vi "wavelength scan_v2.0.vi"() -> ()   [LabVIEW 2012]
panel:
  out "HSRLTEC_offset":dbl=0.01321159999999999 format="%#.4g"
  in  "HSRL_offset":dbl=0.0132 format="%.4g"
  out "Readings":T1={"Pro8000"=TRUE, "WV OnLine TEC"=23.1576786, "WV Online TEC"=TRUE, "WV Online LD"=0.175435558, "WV Online LD"=TRUE, "WV Offline TEC"=29.527338, "WV Offline TEC"=TRUE, "WV Offline LD"=0.175292984, "WV Offline LD"=TRUE, "WV EtalonTEC"=31.6442299, "WV Etalon TEC"=TRUE, "HSRL Etalon TEC"=25.9487457, "HSRL Etalon TEC"=TRUE, "HSRL TEC"=14.2976322, "HSRL TEC "=TRUE, "HSRL LD"=0.160083994, "HSRL LD"=TRUE} {"HSRL LD" format="%.3p"; "HSRL TEC" format="%.3g"; "WV Offline LD" format="%.3p"; "WV Online LD" format="%.3p"; "HSRL Etalon TEC" format="%.3g"; "WV EtalonTEC" format="%.3g"; "WV Offline TEC" format="%.3g"; "WV OnLine TEC" format="%.3g"}
  in  "Settings":T2={"Module"=enum."HSRL TEC", "WV Online TEC"=23.15274999999951, "WV Online LD"=0.175, "WV Offline TEC"=29.514, "WV Offline LD"=0.175, "WV Etalon TEC"=30.61, "HSRL Etalon TEC"=25.954, "HSRL TEC"=14.022, "HSRL LD"=0.16} {"HSRL LD" min=0.0 max=0.18 step=0.001 format="%.3p"; "HSRL TEC" min=14.0 max=28.0 step=0.1 format="%.3g"; "WV Offline LD" min=0.0 max=0.18 step=0.001 format="%.3p"; "WV Online LD" min=0.0 max=0.18 step=0.001 format="%.3p"; "HSRL Etalon TEC" format="%.2g"; "WV Etalon TEC" format="%.2g"; "WV Offline TEC" min=16.0 max=30.0 step=0.1 format="%.3g"; "WV Online TEC" min=14.0 max=28.0 step=0.1 format="%.3g"}
  in  "channel\n0 WV online,\n1, WVoffline\n2, HSRL":i32=2
  out "Power Chart":dbl(graph)=0.0001022
  in  "range (0=auto)":i32
  in  "wavelength":i32=4
  in  "filter (0=out)":i32
  out "OfflineTEC_offset":dbl=0.013673700000001787 format="%#.4g"
  out "OnLineTEC_offset":dbl=0.007064800000488702 format="%.4g"
  in  "WV OnlineTEC_offset":dbl format="%.4g"
  in  "WV OfflineTEC_offset":dbl format="%.4g"
  out "Lambda Read (nm)":dbl=780.2608711081949 format="%.5f"
  out "Wavelength Lock":bool=TRUE
  out "XY Graph":cluster{"Y":dbl[], "Y":dbl[]}[](graph)
  out "Power (W)":dbl=0.0001022 format="%.3p"
  out "OphirPM":T3={"Ophir-Ref"=refnum, "Ophir-Device"=1000, "Ophir-Channel"=0}
  out "Waveform Chart":dbl(graph)=780.2608711081949
  in  "Lambda Step (nm)":dbl=5e-05 format="%.5f"
  in  "Lambda Stop (nm)":dbl=780.261 format="%.5f"
  in  "Lambda Start (nm)":dbl=780.231 format="%.5f"
  in  "step_size":dbl=0.0015 format="%#_6p"
  in  "Device In":refnum<visa-resource-name>="GPIB0::10::INSTR"
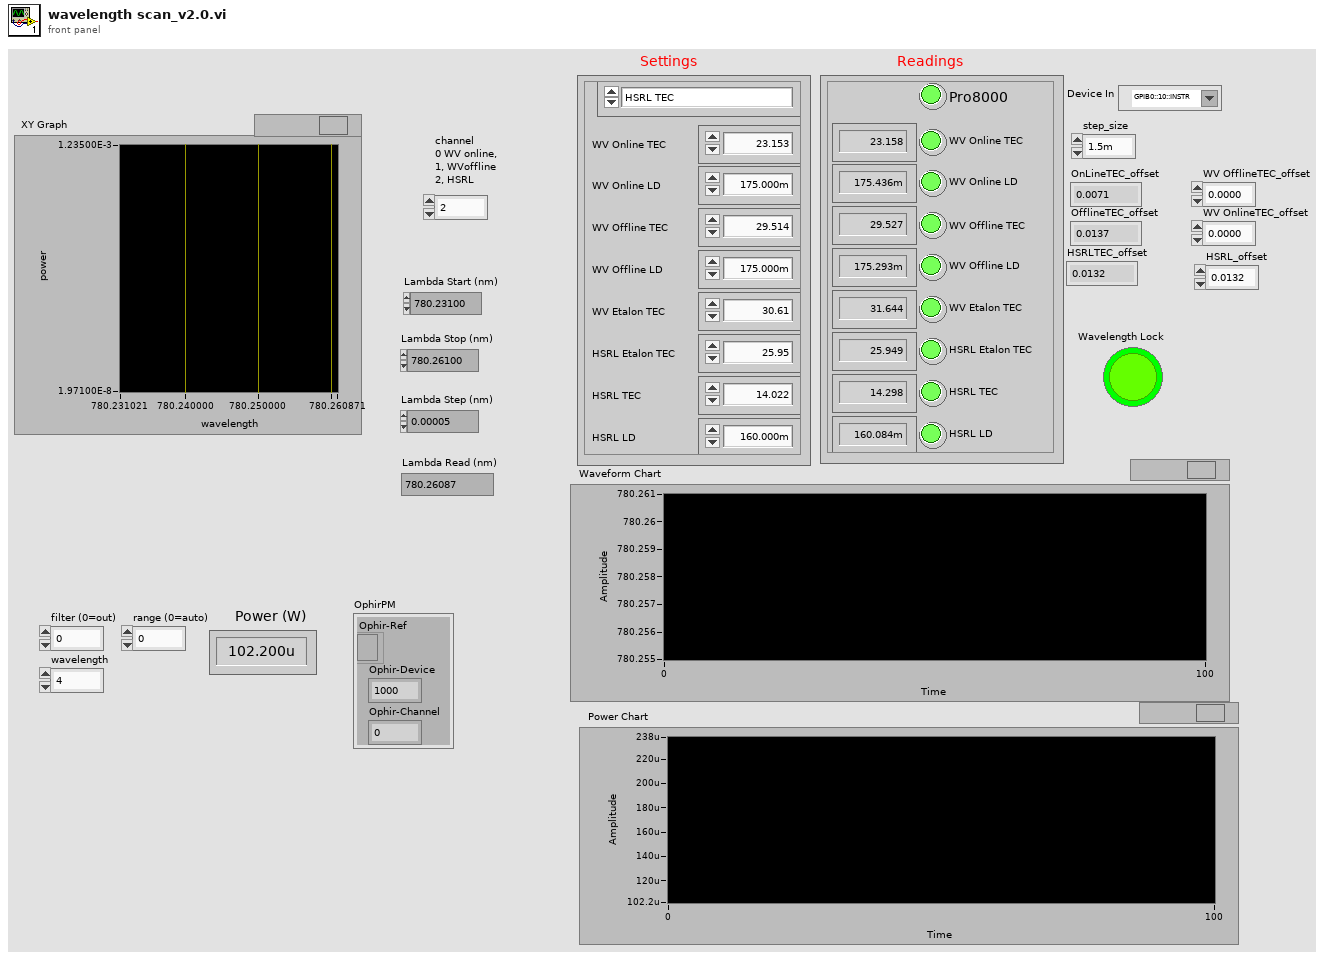
[diagram p1: front panel]
types:
  T1 = cluster{"Pro8000":bool, "WV OnLine TEC":dbl, "WV Online TEC":bool, "WV Online LD":dbl, "WV Online LD":bool, "WV Offline TEC":dbl, "WV Offline TEC":bool, "WV Offline LD":dbl, "WV Offline LD":bool, "WV EtalonTEC":dbl, "WV Etalon TEC":bool, "HSRL Etalon TEC":dbl, "HSRL Etalon TEC":bool, "HSRL TEC":dbl, "HSRL TEC ":bool, "HSRL LD":dbl, "HSRL LD":bool}
  T2 = cluster{"Module":enum16{"WV Online TEC", "WV Online LD", "WV Offline TEC", "WV Offline LD", "WV Etalon TEC", "HSRL Etalon TEC", "HSRL TEC", "HSRL LD"}, "WV Online TEC":dbl, "WV Online LD":dbl, "WV Offline TEC":dbl, "WV Offline LD":dbl, "WV Etalon TEC":dbl, "HSRL Etalon TEC":dbl, "HSRL TEC":dbl, "HSRL LD":dbl}
  T3 = cluster{"Ophir-Ref":refnum<k7>, "Ophir-Device":i32, "Ophir-Channel":i32}
  T4 = enum16{"WV Online TEC", "WV Online LD", "WV Offline TEC", "WV Offline LD", "WV Etalon TEC", "HSRL Etalon TEC", "HSRL TEC", "HSRL LD"}
  T5 = enum16{"Open_TL", "Close_TL", "Verify_ID", "TEC_Sensor", "SET", "READ", "ON", "OFF", "Set_Limits", "Read_Limits", "Enable_Status", "Read_Status"}
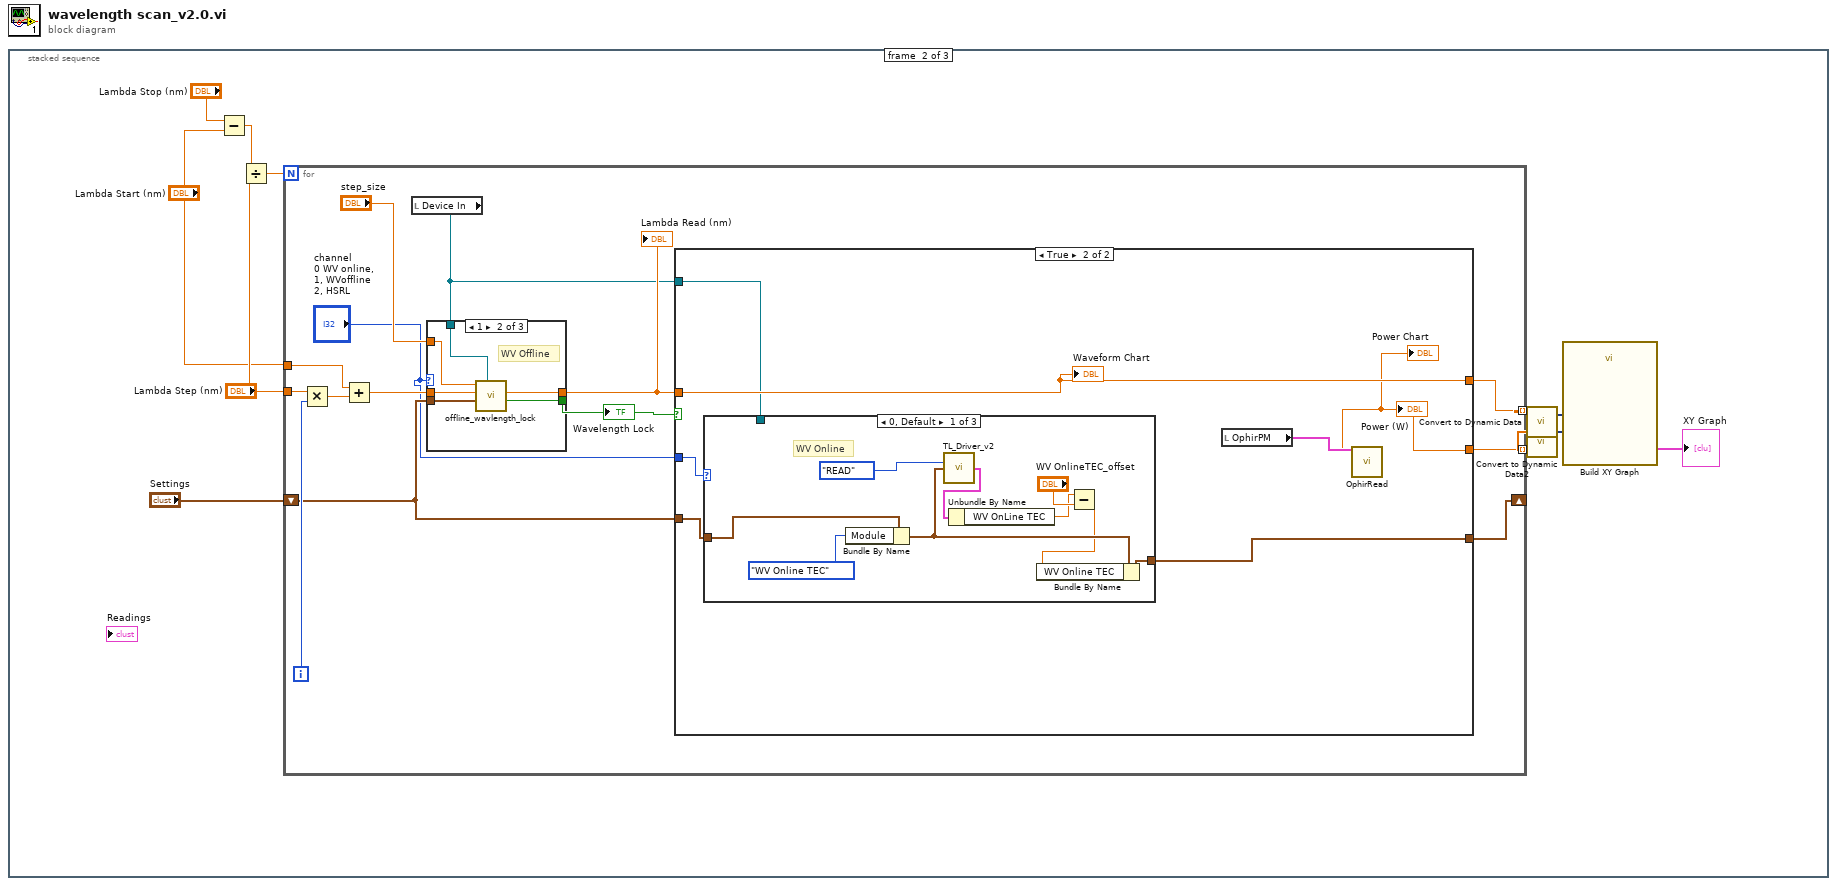
[diagram p0: block diagram]
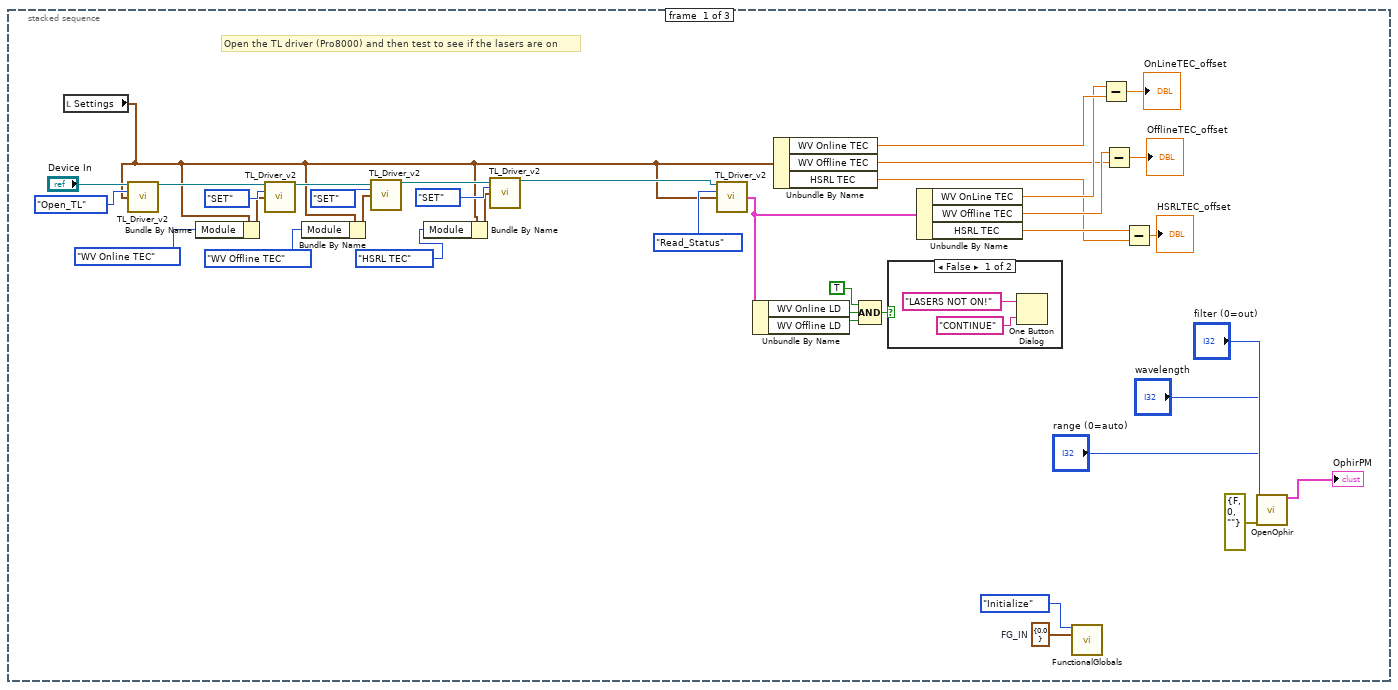
[diagram p2: hidden frame]
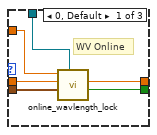
[diagram p4: hidden frame]
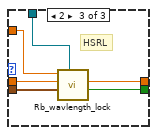
[diagram p5: hidden frame]
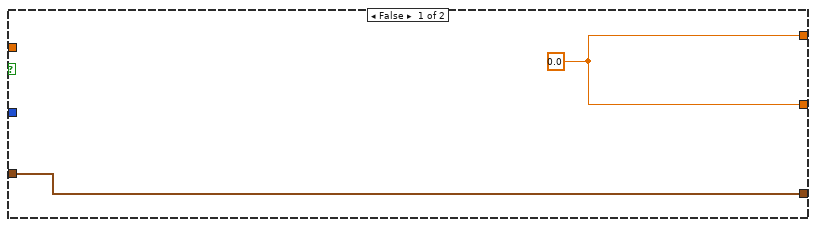
[diagram p6: hidden frame]
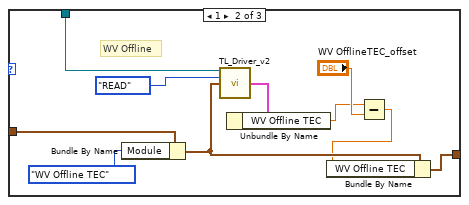
[diagram p7: hidden frame]
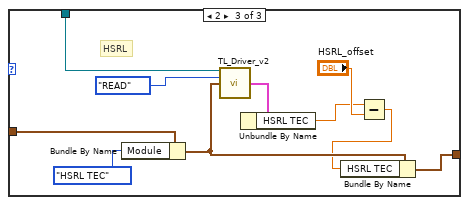
[diagram p8: hidden frame]
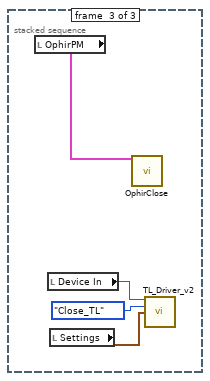
[diagram p9: hidden frame]
diagram:
  n1 = stacked-sequence {
    frame #0 {
      w29 = cluster{"PowerIn":dbl} {"PowerIn"=0.0}  # FG_IN
      # "Open the TL driver (Pro8000) and then test to see if the lasers are on"
      n2 = local read "Settings"() -> (w5:T2)
      n3 = call "TL_Driver_v2.vi"("Device In"="Device In", "Commands"=T5."Open_TL", "Settings"=w5) -> ("Device Out"=w25:refnum<visa-resource-name>)  [unwired: 9 in, 3 out]
      n4 = Bundle By Name(cluster=w5, "Module"=T4."WV Online TEC") -> (w23:T2)
      n5 = call "TL_Driver_v2.vi"("Device In"=w25, "Commands"=T5."SET", "Settings"=w23) -> ("Device Out"=w21:refnum<visa-resource-name>)  [unwired: 9 in, 3 out]
      n6 = Bundle By Name(cluster=w5, "Module"=T4."WV Offline TEC") -> (w22:T2)
      n7 = call "TL_Driver_v2.vi"("Device In"=w21, "Commands"=T5."SET", "Settings"=w22) -> ("Device Out"=w9:refnum<visa-resource-name>)  [unwired: 9 in, 3 out]
      n8 = Bundle By Name(cluster=w5, "Module"=T4."HSRL TEC") -> (w4:T2)
      n9 = call "TL_Driver_v2.vi"("Device In"=w9, "Commands"=T5."SET", "Settings"=w4) -> ("Device Out"=w8:refnum<visa-resource-name>)  [unwired: 9 in, 3 out]
      n10 = call "TL_Driver_v2.vi"("Device In"=w8, "Commands"=T5."Read_Status", "Settings"=w5) -> ("Readings"=w15:T1)  [unwired: 9 in, 3 out]
      n11 = Unbundle By Name(w15) -> ("WV Online LD"=w36:bool, "WV Offline LD"=w35:bool)
      n12 = Unbundle By Name(w5) -> ("WV Online TEC"=w19:dbl, "WV Offline TEC"=w16:dbl, "HSRL TEC"=w2:dbl)
      n13 = Compound Arithmetic op=AND(TRUE, w36, w35) -> (w37:bool)
      n14 = case shown="False" w37 {
        frame False {
          n15 = One Button Dialog(message="LASERS NOT ON!", button name ("OK")="CONTINUE") -> ()  [unwired: 1 out]
        }
        frame True {
        }
      }
      n16 = Unbundle By Name(w15) -> ("WV OnLine TEC"=w18:dbl, "WV Offline TEC"=w17:dbl, "HSRL TEC"=w3:dbl)
      n17 = call "FunctionalGlobals.vi"("FG_Control"=enum16{"Initialize", "PowerRead", "PowerWrite"}."Initialize", "FG_IN"=w29) -> ()  [unwired: 13 in, 1 out]
      n18 = Subtract(x=w18, y=w19) -> (x-y=→"OnLineTEC_offset":dbl)
      n19 = Subtract(x=w17, y=w16) -> (x-y=→"OfflineTEC_offset":dbl)
      n20 = Subtract(x=w3, y=w2) -> (x-y=→"HSRLTEC_offset":dbl)
      n21 = call "OpenOphir.vi"("filter (0=out)"="filter (0=out)", "wavelength"="wavelength", "range (0=auto)"="range (0=auto)", "error in (no error)"=errorcluster {"status"=FALSE, "code"=0, "source"=""}) -> ("OphirPM"=→"OphirPM":T3)  [unwired: 10 in, 1 out]
    }
    frame #1 {
      n22 = Subtract(x="Lambda Stop (nm)", y="Lambda Start (nm)") -> (x-y=w51:dbl)
      n23 = Divide(x=w51, y="Lambda Step (nm)") -> (x/y=w50:dbl)
      n24 = for {
        N: w50 -> [_]
        tunnel: "Lambda Step (nm)" -> [w64]
        tunnel: "Lambda Start (nm)" -> [w63]
        tunnel: [w59] -> w45 mode=indexing
        tunnel: [w58] -> w43 mode=indexing
        shift-right: [w55] -> _
        shift-left: "Settings" -> [w53]
        i -> [w65]
        n25 = Multiply(x=w64, y=w65) -> (x*y=w62:dbl)
        n26 = Add(x=w63, y=w62) -> (x+y=w61:dbl)
        n27 = local read "Device In"() -> (w54:refnum<visa-resource-name>)
        n28 = case shown="1" "channel\n0 WV online,\n1, WVoffline\n2, HSRL" {
          tunnel: w61 -> [w71 w75 w81]
          tunnel: w54 -> [w70 w76 w82]
          tunnel: w53 -> [w69 w74 w80]
          tunnel: [w68 w73 w79] -> w57
          tunnel: [w67 w72 w78] -> w56
          tunnel: "step_size" -> [w66 w77 w83]
          frame 0, Default {
            # "WV Online"
            n29 = call "online_wavlength_lock.vi"("Device"=w70, "Settings"=w69, "Lambda On Set (nm)"=w71, "step_size"=w66) -> ("Wavelength Lock Online"=w68:bool, "Lambda On Read (nm)"=w67:dbl)  [unwired: 3 in]
          }
          frame 1 {
            # "WV Offline"
            n30 = call "offline_wavlength_lock.vi"("Device"=w76, "Settings"=w74, "Lambda Off Set (nm)"=w75, "step_size"=w77) -> ("Wavelength Lock Offline"=w73:bool, "Lambda Off Read (nm)"=w72:dbl)  [unwired: 3 in]
          }
          frame 2 {
            # "HSRL"
            n31 = call "Rb_wavlength_lock.vi"("Device"=w82, "Settings"=w80, "Lambda Set (nm)"=w81, "step_size"=w83) -> ("Wavelength Lock"=w79:bool, "Lambda Read (nm)"=w78:dbl)  [unwired: 3 in]
          }
        }
        "Wavelength Lock" <- w57
        "Lambda Read (nm)" <- w56
        n32 = case shown="True" w57 {
          tunnel: w56 -> [_ w91]
          tunnel: [w85 w91] -> w59
          tunnel: [w85 w86] -> w58
          tunnel: [w84 w87] -> w55
          tunnel: w54 -> [_ w90]
          tunnel: w53 -> [w84 w89]
          tunnel: "channel\n0 WV online,\n1, WVoffline\n2, HSRL" -> [_ w88]
          frame False {
            w85 = 0.0
          }
          frame True {
            n33 = case shown="0, Default" w88 {
              tunnel: w90 -> [_ w110 w120]
              tunnel: w89 -> [w101 w109 w119]
              tunnel: [w97 w106 w116] -> w87
              frame 0, Default {
                # "WV Online"
                n34 = Bundle By Name(cluster=w101, "Module"=T4."WV Online TEC") -> (w98:T2)
                n35 = call "TL_Driver_v2.vi"("Commands"=T5."READ", "Settings"=w98) -> ("Readings"=w99:T1)  [unwired: 10 in, 3 out]
                n36 = Unbundle By Name(w99) -> ("WV OnLine TEC"=w95:dbl)
                n37 = Subtract(x=w95, y="WV OnlineTEC_offset") -> (x-y=w94:dbl)
                n38 = Bundle By Name(cluster=w98, "WV Online TEC"=w94) -> (w97:T2)
              }
              frame 1 {
                # "WV Offline"
                n39 = Bundle By Name(cluster=w109, "Module"=T4."WV Offline TEC") -> (w107:T2)
                n40 = call "TL_Driver_v2.vi"("Device In"=w110, "Commands"=T5."READ", "Settings"=w107) -> ("Readings"=w108:T1)  [unwired: 9 in, 3 out]
                n41 = Unbundle By Name(w108) -> ("WV Offline TEC"=w104:dbl)
                n42 = Subtract(x=w104, y="WV OfflineTEC_offset") -> (x-y=w103:dbl)
                n43 = Bundle By Name(cluster=w107, "WV Offline TEC"=w103) -> (w106:T2)
              }
              frame 2 {
                # "HSRL"
                n44 = Bundle By Name(cluster=w119, "Module"=T4."HSRL TEC") -> (w117:T2)
                n45 = call "TL_Driver_v2.vi"("Device In"=w120, "Commands"=T5."READ", "Settings"=w117) -> ("Readings"=w118:T1)  [unwired: 9 in, 3 out]
                n46 = Unbundle By Name(w118) -> ("HSRL TEC"=w114:dbl)
                n47 = Subtract(x=w114, y="HSRL_offset") -> (x-y=w113:dbl)
                n48 = Bundle By Name(cluster=w117, "HSRL TEC"=w113) -> (w116:T2)
              }
            }
            n49 = local read "OphirPM"() -> (w92:T3)
            n50 = call "OphirRead.vi"("OphirPM"=w92) -> ("Power (W)"=w86:dbl)  [unwired: 12 in, 2 out]
            "Power (W)" <- w86
            "Power Chart" <- w86
            "Waveform Chart" <- w91
          }
        }
      }
      n51 = call "Convert to Dynamic Data"("Array"=w45) -> ("Dynamic Data Type"=w44:dynamicdata)  [unwired: 3 in]
      n52 = call "Convert to Dynamic Data2"("Array"=w43) -> ("Dynamic Data Type"=w42:dynamicdata)  [unwired: 3 in]
      n53 = call "Build XY Graph"("Y Input"=w42, "X Input"=w44) -> ("XY Graph"=→"XY Graph":cluster{"Y":dbl[], "Y":dbl[]}[])  [unwired: 3 in, 6 out]
    }
    frame #2 {
      n54 = local read "OphirPM"() -> (w125:T3)
      n55 = local read "Device In"() -> (w122:refnum<visa-resource-name>)
      n56 = local read "Settings"() -> (w123:T2)
      n57 = call "OphirClose.vi"("OphirPM"=w125) -> ()  [unwired: 18 in, 1 out]
      n58 = call "TL_Driver_v2.vi"("Device In"=w122, "Commands"=T5."Close_TL", "Settings"=w123) -> ()  [unwired: 9 in, 4 out]
    }
  }
